vi "matrici_v9.vi"() -> ()   [LabVIEW 2009]
panel:
  out "Elementul selectat":u8=64
  in  "Linia":u8(slide)=3 scale=0.0..6.0
  in  "Coloana":u8(slide)=2 scale=0.0..4.0
  in  "stop":bool
  in  "Valoarea maxima":dbl(knob)=76.8880655921393 scale=0.0..100.0
  out "Matrice numerica 7X5":u8[][](array[numeric])=[[2, 53, 47, 41, 61], [33, 68, 23, 65, 14], [2, 47, 29, 41, 60], [33, 30, 64, 29, 36], [9, 13, 46, 5, 56], [67, 3, 16, 49, 31], [32, 69, 11, 33, 32]]
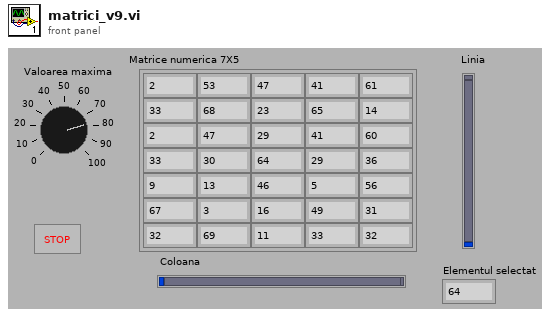
[diagram p1: front panel]
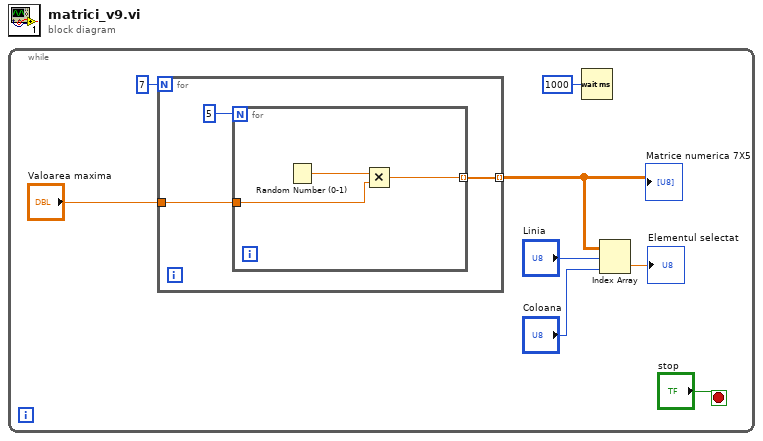
[diagram p0: block diagram]
diagram:
  n1 = while {
    stop <- "stop" stop-if-true
    n2 = for {
      N: 7 -> [_]
      tunnel: "Valoarea maxima" -> [w10]
      tunnel: [w9] -> w4 mode=indexing
      n3 = for {
        N: 5 -> [_]
        tunnel: [w13] -> w9 mode=indexing
        tunnel: w10 -> [w12]
        n4 = Random Number (0-1)() -> (number: 0 to 1=w14:dbl)
        n5 = Multiply(x=w14, y=w12) -> (x*y=w13:dbl)
      }
    }
    "Matrice numerica 7X5" <- w4
    n6 = Wait (ms)(milliseconds to wait=u32 1000) -> ()  [unwired: 1 out]
    n7 = Index Array(array=w4, index (row)="Linia", index (col)="Coloana") -> (element=→"Elementul selectat":dbl)
  }
